vi "Pockels Cal_Update single cal core.vi"(10 "New cal section":string[][](array[string])=[["Cal Wavelength", "", "", ""], ["820", "", "", ""], ["Prism 1:", "2039", "", ""], ["Prism 2:", "1953", "", ""], ["Pockels bias:", "199", "", ""], ["Zoom:", "12", "", ""], ["Dwell time:", "0.4", "", ""], ["Cal subset indexes", "", "", ""], ["0", "15", "", ""], ["Cal data", "", "", ""], ["Pockels V", "No objective", "Objective B", "New Objective"], ["0", "0", "7", "1"], ["0.1", "2.8", "7", "1"], ["0.2", "9.8", "7", "1"], ["0.3", "21.4", "", "1"], ["0.4", "37.1", "", ""], ["0.5", "56.1", "", ""], ["0.6", "77.7", "", ""], ["0.7", "101", "", ""], ["0.8", "125", "", ""], ["0.9", "148", "", ""], ["1", "169", "", ""], ["1.1", "188", "", ""], ["1.2", "204", "", ""], ["1.3", "215", "", ""], ["1.4", "222", "", ""], ["1.5", "225", "", ""], ["1.6", "222", "", ""], ["1.7", "214", "", ""], ["1.8", "202", "", ""], ["1.9", "187", "", ""], ["2", "152", "", ""]], 11 "Loaded cal section":string[][](array[string])=[["Cal Wavelength", "", "", ""], ["820", "", "", ""], ["Prism 1:", "2039", "", ""], ["Prism 2:", "1953", "", ""], ["Pockels bias:", "199", "", ""], ["Zoom:", "12", "", ""], ["Dwell time:", "0.4", "", ""], ["Cal subset indexes", "", "", ""], ["0", "15", "", ""], ["Cal data", "", "", ""], ["Pockels V", "No objective", "Objective A", "Objective B"], ["0", "0", "", "1"], ["0.1", "2.8", "", "2"], ["0.2", "9.8", "", "3"], ["0.3", "21.4", "", "4"], ["0.4", "37.1", "", "5"], ["0.5", "56.1", "", "6"], ["0.6", "77.7", "", "7"], ["0.7", "101", "", ""], ["0.8", "125", "", ""], ["0.9", "148", "", ""], ["1", "169", "", ""], ["1.1", "188", "", ""], ["1.2", "204", "", ""], ["1.3", "215", "", ""], ["1.4", "222", "", ""], ["1.5", "225", "", ""], ["1.6", "222", "", ""], ["1.7", "214", "", ""], ["1.8", "202", "", ""], ["1.9", "187", "", ""], ["2", "152", "", ""]]) -> (3 "Updated cal section":string[][](array[string]))   [LabVIEW 2020]
uses:
  gl_Calibration globals.vi
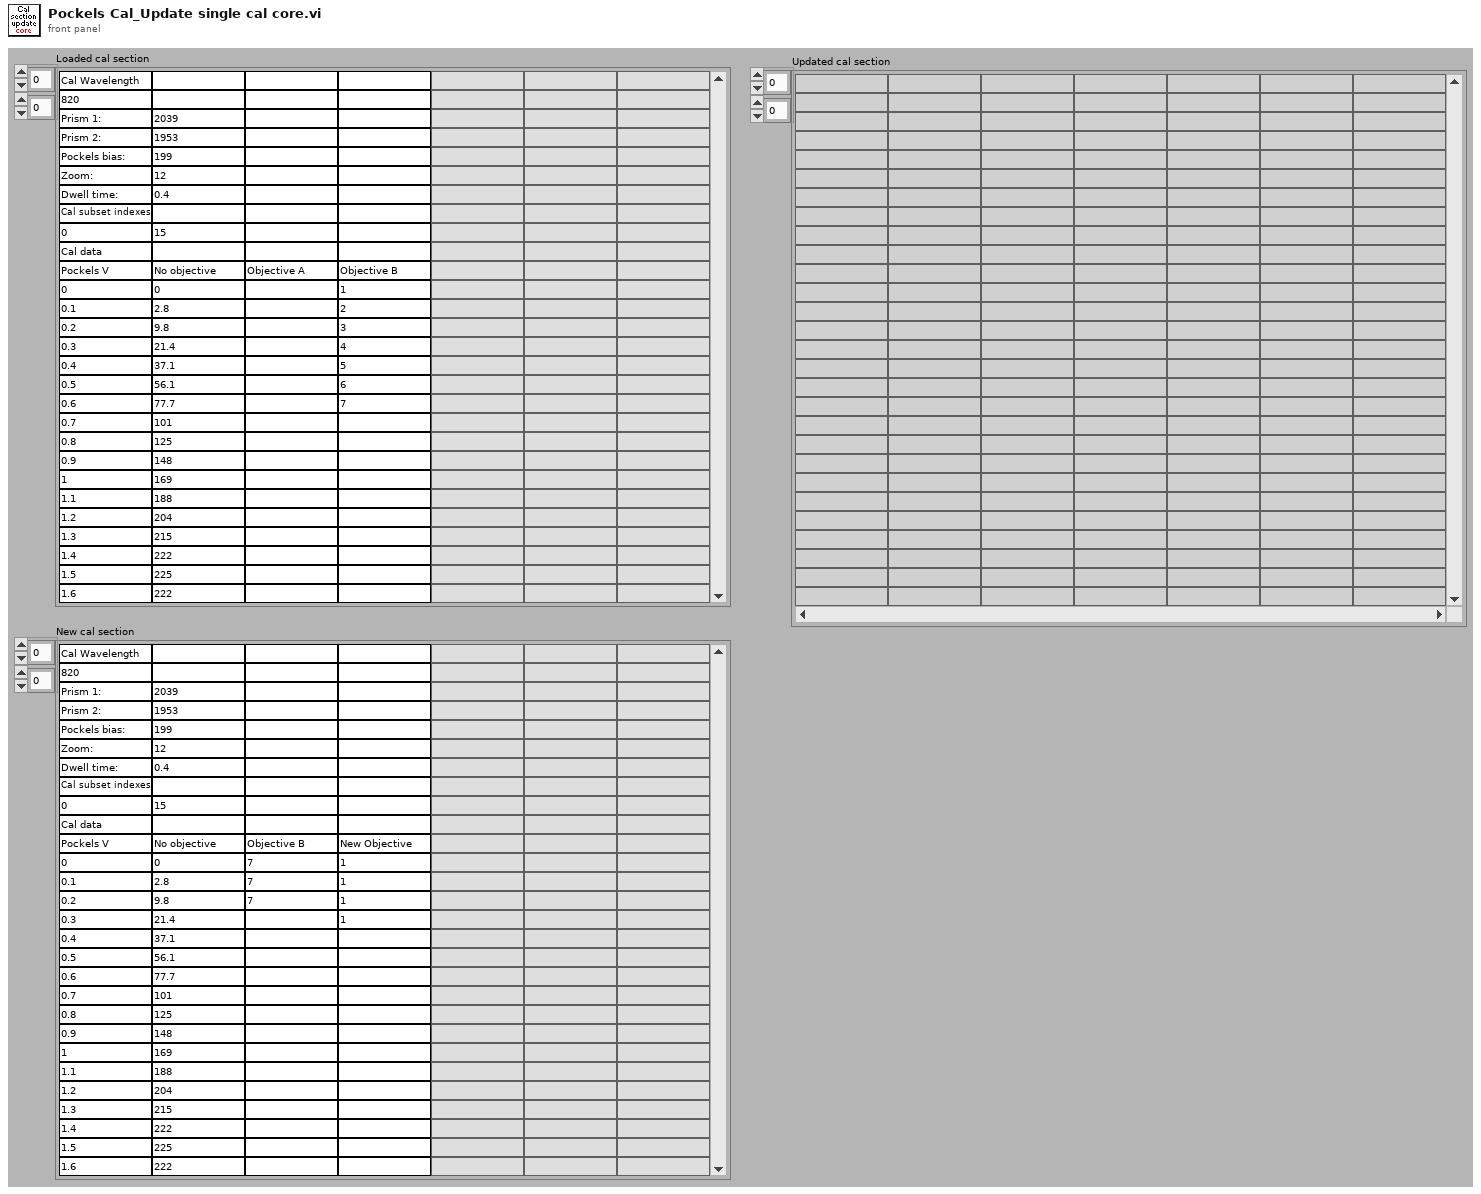
[diagram p1: front panel]
types:
  T1 = typedef "Pockels cal conditions row indexes cluster.ctl" = cluster{"Wavelength index (in column zero)":i32, "Zoom index":i32, "Dwell time (us) index":i32, "Pockels bias index":i32, "Prism 1 index":i32, "Prism 2 index":i32, "Laser power index":i32}
  T2 = typedef "Pockels cal conditions cluster.ctl" = cluster{"Wavelength":u16, "Zoom":u8, "Dwell time (us)":dbl, "Pockels bias":i16, "Prism 1":u16, "Prism 2":u16, "Laser power during pockels cal (mW)":u16}
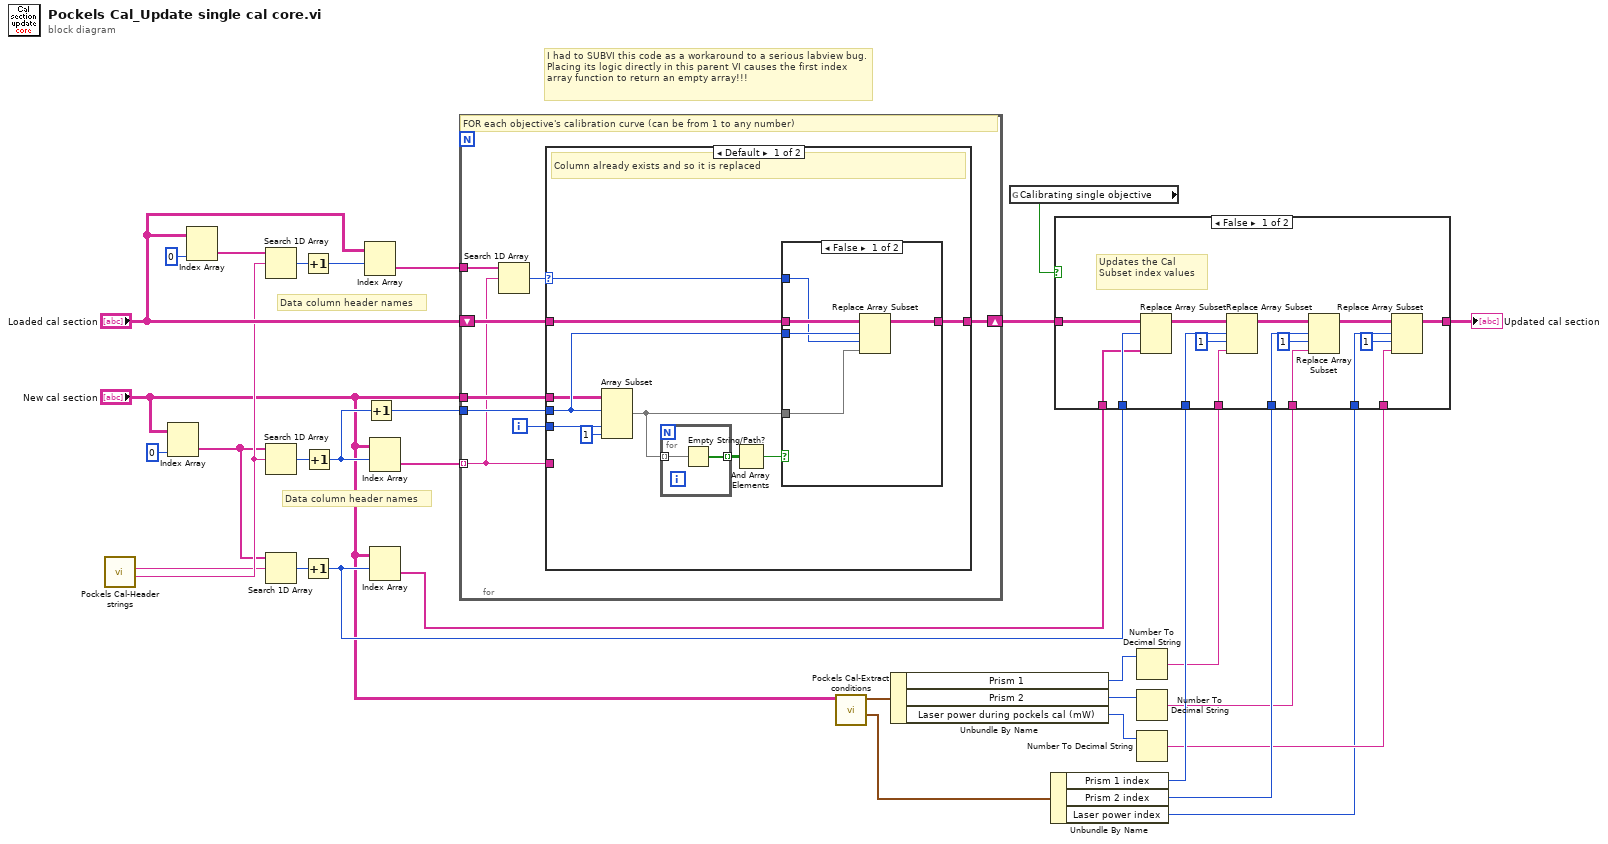
[diagram p0: block diagram]
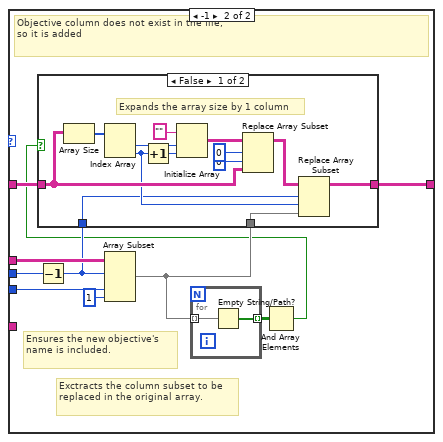
[diagram p4: hidden frame]
diagram:
  # "Data column header names"
  # "Data column header names"
  # "I had to SUBVI this code as a workaround to a serious labview bug. Placing its logic directly in this parent VI causes the first index array function to return an empty array!!!"
  n1 = call "Pockels Cal-Header strings.vi"() -> ("Cal data header string"=w21:string, "Cal subset indexes header string"=w20:string)  [unwired: 9 in, 1 out]
  n2 = Index Array(array="New cal section", index (col)=0 ("disabled index (col)")) -> (element=w18:string[])  [unwired: 1 in]
  n3 = Index Array(array="Loaded cal section", index (col)=0 ("disabled index (col)")) -> (element=w25:string[])  [unwired: 1 in]
  n4 = Search 1D Array(1D array=w25, element=w21) -> (index of element=w26:i32)  [unwired: 1 in]
  n5 = Search 1D Array(1D array=w18, element=w21) -> (index of element=w31:i32)  [unwired: 1 in]
  n6 = Search 1D Array(1D array=w18, element=w20) -> (index of element=w19:i32)  [unwired: 1 in]
  n7 = Increment(x=w26) -> (x+1=w28:i32)
  n8 = Increment(x=w19) -> (x+1=w16:i32)
  n9 = Increment(x=w31) -> (x+1=w23:i32)
  n10 = Index Array(array="Loaded cal section", index (row)=w28) -> (element=w24:string[])  [unwired: 1 in]
  n11 = Increment(x=w23) -> (x+1=w22:i32)
  n12 = Index Array(array="New cal section", index (row)=w23) -> (element=w29:string[])  [unwired: 1 in]
  n13 = Index Array(array="New cal section", index (row)=w16) -> (element=w15:string[])  [unwired: 1 in]
  n14 = for {
    tunnel: w22 -> [w40]
    tunnel: "New cal section" -> [w38]
    shift-right: [w36] -> w17
    shift-left: "Loaded cal section" -> [w37]
    tunnel: w29 -> [w33] mode=indexing
    tunnel: w24 -> [w35]
    i -> [w39]
    # "FOR each objective's calibration curve (can be from 1 to any number)"
    n15 = Search 1D Array(1D array=w35, element=w33) -> (index of element=w34:i32)  [unwired: 1 in]
    n16 = case shown="Default" w34 {
      selector: w34 -> [w44 _]
      tunnel: w40 -> [w50 w68]
      tunnel: w39 -> [w49 w67]
      tunnel: w38 -> [w48 w66]
      tunnel: w37 -> [w47 w63]
      tunnel: [w46 w65] -> w36
      tunnel: w33 -> [_ _]
      frame Default {
        # "Column already exists and so it is replaced"
        n17 = Array Subset "Array Subset"(array=w48, index (row)=w50, index (col)=w49, length (col)=1 ("length")) -> (w43:string[][])  [unwired: 1 in]
        n18 = for {
          tunnel: w43 -> [w52] mode=indexing
          tunnel: [w51] -> w42 mode=indexing
          n19 = Empty String/Path?(string/path=w52) -> (empty?=w51:bool[])
        }
        n20 = And Array Elements(Boolean array=w42) -> (logical AND=w41:bool)
        n21 = case shown="False" w41 {
          tunnel: w50 -> [w57 _]
          tunnel: w47 -> [w56 w58]
          tunnel: [w55 w58] -> w46
          tunnel: w44 -> [w54 _]
          tunnel: w43 -> [w53 _]
          frame False {
            n22 = Replace Array Subset "Replace Array Subset"(array=w56, new element=w53, index (row)=w57, index (col)=w54) -> (w55:string[][])
          }
          frame True {
            # "Fail-safe\npreventing adding\nempty data arrays"
          }
        }
      }
      frame -1 {
        # "Exctracts the column subset to be replaced in the original array."
        # "Objective column does not exist in the file,\nso it is added"
        # "Ensures the new objective's name is included."
        n23 = Decrement(x=w68) -> (x-1=w62:i32)
        n24 = Array Subset "Array Subset"(array=w66, index (row)=w62, index (col)=w67, length (col)=1 ("length")) -> (w60:string[][])  [unwired: 1 in]
        n25 = for {
          tunnel: w60 -> [w84] mode=indexing
          tunnel: [w83] -> w61 mode=indexing
          n26 = Empty String/Path?(string/path=w84) -> (empty?=w83:bool[])
        }
        n27 = And Array Elements(Boolean array=w61) -> (logical AND=w59:bool)
        n28 = case shown="False" w59 {
          tunnel: [w81 w82] -> w65
          tunnel: w63 -> [w75 w82]
          tunnel: w62 -> [w70 _]
          tunnel: w60 -> [w69 _]
          frame False {
            # "Expands the array size by 1 column"
            n29 = Array Size(array=w75) -> (size(s)=w80:i32[])
            n30 = Index Array(array=w80) -> (element #1=w79:i32, element #2=w71:i32)  [unwired: 2 in]
            n31 = Increment(x=w71) -> (x+1=w72:i32)
            n32 = Initialize Array("" ("element"), w79, w72) -> (w77:string[][])
            n33 = Replace Array Subset "Replace Array Subset"(array=w77, new element=w75, index (row)=0, index (col)=0 ("disabled index (col)")) -> (w73:string[][])
            n34 = Replace Array Subset(array=w73, new element=w69, index (row)=w70, index (col)=w71) -> (w81:string[][])
          }
          frame True {
            # "Fail-safe\npreventing adding\nempty data arrays"
          }
        }
      }
    }
  }
  n35 = call "Pockels Cal-Extract conditions.vi"("Pockels Cal table (full)"="New cal section") -> ("Pockels cal conditions row index"=w9:T1, "Pockels cal conditions"=w13:T2)  [unwired: 8 in, 1 out]
  n36 = Unbundle By Name(w13) -> ("Prism 1"=w12:u16, "Prism 2"=w11:u16, "Laser power during pockels cal (mW)"=w10:u16)
  n37 = global read "gl_Calibration globals.vi" "Calibrating single objective"() -> (w1:bool)
  n38 = Unbundle By Name(w9) -> ("Prism 1 index"=w8:i32, "Prism 2 index"=w6:i32, "Laser power index"=w2:i32)
  n39 = Number To Decimal String(number=w12) -> (decimal integer string=w7:string)  [unwired: 1 in]
  n40 = Number To Decimal String(number=w11) -> (decimal integer string=w5:string)  [unwired: 1 in]
  n41 = Number To Decimal String(number=w10) -> (decimal integer string=w3:string)  [unwired: 1 in]
  n42 = case shown="False" w1 {
    tunnel: w17 -> [w100 w101]
    tunnel: w16 -> [w99 _]
    tunnel: w15 -> [w98 _]
    tunnel: w8 -> [w96 _]
    tunnel: w7 -> [w94 _]
    tunnel: w6 -> [w91 _]
    tunnel: w5 -> [w90 _]
    tunnel: [w87 w101] -> w4
    tunnel: w3 -> [w86 _]
    tunnel: w2 -> [w85 _]
    frame False {
      # "Updates the Cal Subset index values"
      n43 = Replace Array Subset(array=w100, new element=w98, index (row)=w99) -> (w97:string[][])  [unwired: 1 in]
      n44 = Replace Array Subset(array=w97, new element=w94, index (row)=w96, index (col)=1 ("disabled index (col)")) -> (w92:string[][])
      n45 = Replace Array Subset(array=w92, new element=w90, index (row)=w91, index (col)=1 ("disabled index (col)")) -> (w88:string[][])
      n46 = Replace Array Subset(array=w88, new element=w86, index (row)=w85, index (col)=1 ("disabled index (col)")) -> (w87:string[][])
    }
    frame True {
      # "Calibrating single objective"
    }
  }
  "Updated cal section" <- w4
